vi "Actor Core.vi"(8 "error in":errorcluster, 11 "Nested in":refnum<class "Timer_Event.lvclass">) -> (0 "error out":errorcluster, 3 "Actor out":refnum<class "Actor.lvclass">)   [LabVIEW 2020, in "Timer_Event.lvlib" / "Timer_Event.lvclass"]
doc: "(<B>Filename</B>: Actor Framework.lvlib:Actor.lvclass:Actor Core.vi)\n\nReceives messages to the actor, reacts to them, and initiates any error handling that may shut the actor down.\n\nDescendant classes may override this VI to append parallel tasks for the actor to complete while it handles messages. Overrides use the Call Parent Method node."
uses:
  Timer_Event.lvclass
  C:/Program Files (x86)/National Instruments/LabVIEW 2020/vi.lib/ActorFramework/Actor/Actor.lvclass
  <vilib>/ActorFramework/Actor/Actor.lvclass
  <vilib>/ActorFramework/Actor/Actor.lvclass/Actor.ctl
  <vilib>/ActorFramework/Message Enqueuer/Message Enqueuer.lvclass/Message Enqueuer.ctl
  Timer_Event.lvclass/Timer_Event.ctl
  <vilib>/ActorFramework/Message Enqueuer/Init from Existing Queue.vi
  <vilib>/ActorFramework/Message Enqueuer/Enqueue.vi
  <vilib>/ActorFramework/Stop Msg/Stop Msg.lvclass
  C:/Program Files (x86)/National Instruments/LabVIEW 2020/vi.lib/ActorFramework/Message/Message.lvclass
  Timer_Event Messages/Start Msg/Start Msg.lvclass
  Timer_Event Messages/Stop_Timer Msg/Stop_Timer Msg.lvclass
  Timer_Event Messages/Get_Timer Msg/Get_Timer Msg.lvclass
  Timer_Event Messages/UpdateTimerToCaller Msg/UpdateTimerToCaller Msg.lvclass
  Timer_Event Messages/Reset_Timer Msg/Reset_Timer Msg.lvclass
  <vilib>/ActorFramework/Message Priority Queue/Priority Enqueue.vi
  <vilib>/ActorFramework/Message Enqueuer/Message Enqueuer.lvclass
panel:
  out "Time (ms)":u32
  out "Running":bool
  in  "Start":bool
  in  "Stop":bool
  in  "Reset":bool
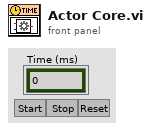
[diagram p1: front panel]
types:
  T1 = cluster{"Stop":refnum<user-event>, "Elapsed Time (ms)":refnum<user-event>, "Running":refnum<user-event>}
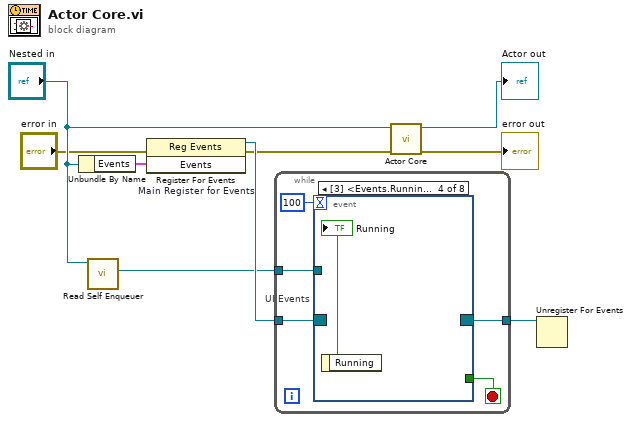
[diagram p0: block diagram]
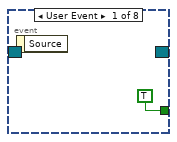
[diagram p2: hidden frame]
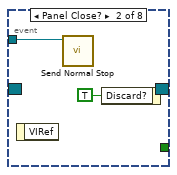
[diagram p3: hidden frame]
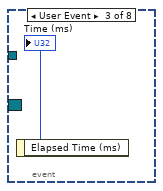
[diagram p4: hidden frame]
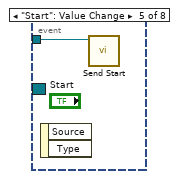
[diagram p5: hidden frame]
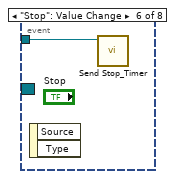
[diagram p6: hidden frame]
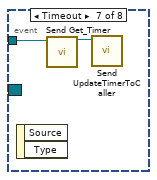
[diagram p7: hidden frame]
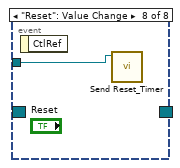
[diagram p8: hidden frame]
diagram:
  n1 = Unbundle By Name("Nested in") -> ("Events"=w6:T1)
  n2 = call <vilib>:"Read Self Enqueuer.vi"("Actor"="Nested in") -> ("Self Enqueuer"=w3:refnum<class "Message Enqueuer.lvclass">)  [unwired: 10 in]
  n3 = register-events "Main Register for Events"(error in="error in", w6) -> (reference out=w7:refnum<event-registration>, error out=w1:errorcluster)  [unwired: 1 in]
  n4 = while {
    tunnel: w7 -> [w14]
    tunnel: [w12] -> w5
    tunnel: w3 -> [w11]
    stop <- w13 stop-if-true
    n5 = event "UI Events" shown="[3] <Events.Running>: User Event" {
      selector: w14 -> [_ _ _ _ _ _ _ _]
      dyn-events: [_ _ _ _ _ _ _ _] -> w12
      timeout: 100 -> [_ _ _ _ _ _ _ _]
      tunnel: [TRUE _ _ _ _ _ _ _] -> w13
      tunnel: w11 -> [_ w16 _ _ w20 w21 w23 w24]
      event User Event {
        n6 = event-data() -> ()  [unwired: 1 in, 1 out]
      }
      event Panel Close? {
        n7 = event-data() -> ()  [unwired: 1 in, 1 out]
        n8 = call <vilib>:"Send Normal Stop.vi"("Message Enqueuer"=w16) -> ()  [unwired: 10 in, 1 out]
        n9 = event-data("Discard?"=TRUE) -> ()  [unwired: 1 in, 1 out]
      }
      event User Event {
        n10 = event-data() -> ("Elapsed Time (ms)"=→"Time (ms)":u32)  [unwired: 1 in]
      }
      event User Event {
        n11 = event-data() -> ("Running"=→"Running":bool)  [unwired: 1 in]
      }
      event "Start": Value Change {
        n12 = event-data() -> ()  [unwired: 1 in, 2 out]
        n13 = call "Send Start.vi"("Message Enqueuer"=w20) -> ()  [unwired: 9 in, 2 out]
      }
      event "Stop": Value Change {
        n14 = event-data() -> ()  [unwired: 1 in, 2 out]
        n15 = call "Send Stop_Timer.vi"("Message Enqueuer"=w21) -> ()  [unwired: 9 in, 2 out]
      }
      event Timeout {
        n16 = event-data() -> ()  [unwired: 1 in, 2 out]
        n17 = call "Send Get_Timer.vi"("Message Enqueuer"=w23) -> ("Message Enqueuer out"=w22:refnum<class "Message Enqueuer.lvclass">)  [unwired: 9 in, 1 out]
        n18 = call "Send UpdateTimerToCaller.vi"("Message Enqueuer"=w22) -> ()  [unwired: 9 in, 2 out]
      }
      event "Reset": Value Change {
        n19 = event-data() -> ()  [unwired: 1 in, 1 out]
        n20 = call "Send Reset_Timer.vi"("Message Enqueuer"=w24) -> ()  [unwired: 9 in, 2 out]
      }
    }
  }
  n21 = call-parent "Actor Core.vi"("error in"=w1, "Actor in"="Nested in") -> ("error out"=→"error out":errorcluster, "Actor out"=→"Actor out":refnum<class "Actor.lvclass">)  [unwired: 8 in]
  n22 = Unregister For Events(event registration refnum=w5) -> ()  [unwired: 1 in, 1 out]
